vi "Read GUID.vi"(8 "error in (no error)":errorcluster, 11 "Rooms Manager Model in":refnum<class "Rooms Manager Model.lvclass">) -> (0 "error out":errorcluster, 2 "GUID":string, 3 "Rooms Manager Model out":refnum<class "Rooms Manager Model.lvclass">)   [LabVIEW 2023, in "Rooms Manager Model.lvlib" / "Rooms Manager Model.lvclass"]
uses:
  Rooms Manager Model.lvclass
  Rooms Manager Model.lvclass/Rooms Manager Model.ctl
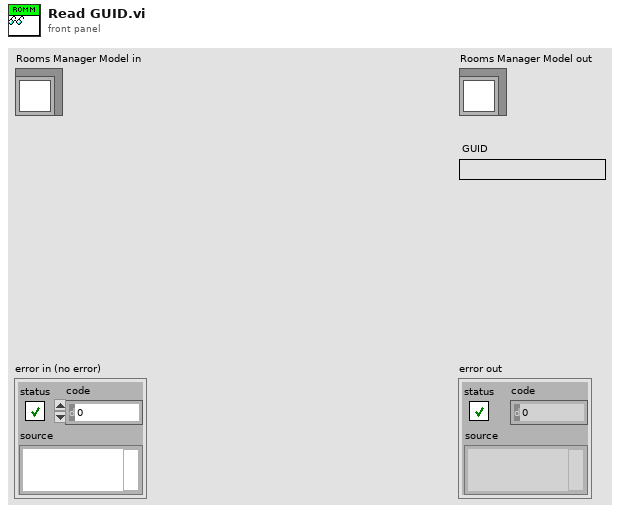
[diagram p1: front panel]
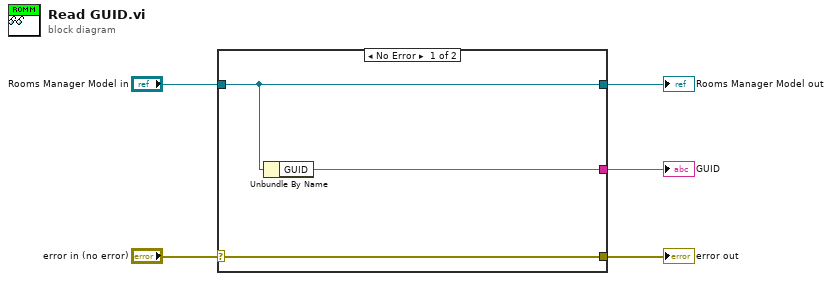
[diagram p0: block diagram]
diagram:
  n1 = case shown="No Error" "error in (no error)" {
    selector: "error in (no error)" -> [w8 w9]
    tunnel: [w8 w9] -> w4
    tunnel: [w7 w10] -> w2
    tunnel: "Rooms Manager Model in" -> [w7 w10]
    tunnel: [w6 _] -> w1
    frame No Error {
      n2 = Unbundle By Name(w7) -> ("GUID"=w6:string)
    }
    frame Error {
    }
  }
  "error out" <- w4
  "Rooms Manager Model out" <- w2
  "GUID" <- w1
